vi "OP500ZP_CLUSTER_OCVACIR.vi"(10 "MESURES_OCVACIR":cluster{string, string, string}, 11 "Tableau 3":string[][](array[string])) -> (2 "Tableau":bool[](array[boolean]), 3 "Tableau 2":string[][](array[string]))   [LabVIEW 2020]
uses:
  VG/PackType.vi
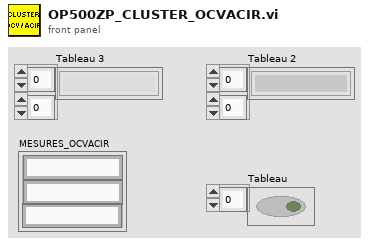
[diagram p1: front panel]
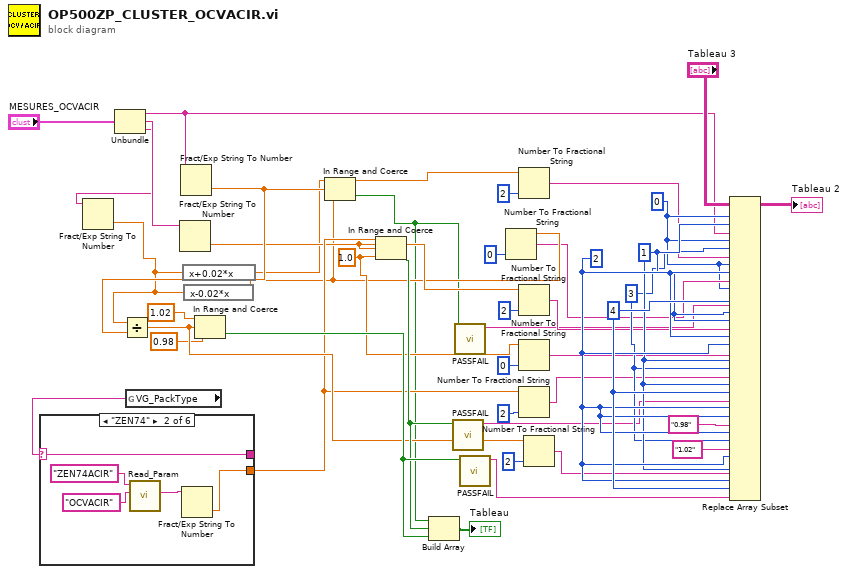
[diagram p0: block diagram]
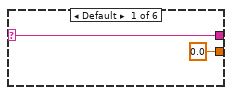
[diagram p2: hidden frame]
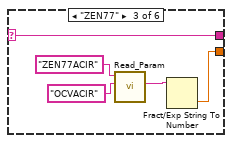
[diagram p3: hidden frame]
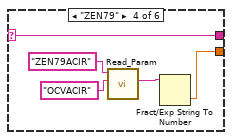
[diagram p4: hidden frame]
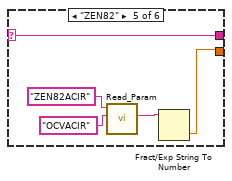
[diagram p5: hidden frame]
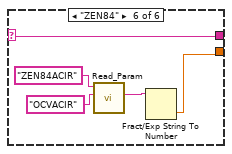
[diagram p6: hidden frame]
diagram:
  w20 = 1.0 ("limite inférieure")
  w37 = 2 ("disabled index (col)")
  w38 = 4 ("disabled index (col)")
  w34 = 3 ("disabled index (col)")
  w35 = 1 ("disabled index (col)")
  w11 = 0 ("index (row)")
  n1 = Unbundle("MESURES_OCVACIR") -> (w4:string, w3:string, w1:string)
  n2 = Fract/Exp String To Number(string=w1) -> (number=w2:dbl)  [unwired: 3 in, 1 out]
  n3 = global read "PackType.vi" "VG_PackType"() -> (w14:string)
  n4 = case shown="\"ZEN74\"" w14 {
    selector: w14 -> [w45 w50 w55 w60 w65 w70]
    tunnel: [w45 w50 w55 w60 w65 w70] -> _
    tunnel: [0.0 ("ZEN84ACIR") w46 w51 w56 w61 w66] -> w23
    frame Default {
    }
    frame "ZEN74" {
      n5 = call "Read_Param.vi"("section"="OCVACIR", "key"="ZEN74ACIR") -> ("str"=w49:string)  [unwired: 5 in, 4 out]
      n6 = Fract/Exp String To Number(string=w49) -> (number=w46:dbl)  [unwired: 3 in, 1 out]
    }
    frame "ZEN77" {
      n7 = call "Read_Param.vi"("section"="OCVACIR", "key"="ZEN77ACIR") -> ("str"=w54:string)  [unwired: 5 in, 4 out]
      n8 = Fract/Exp String To Number(string=w54) -> (number=w51:dbl)  [unwired: 3 in, 1 out]
    }
    frame "ZEN79" {
      n9 = call "Read_Param.vi"("section"="OCVACIR", "key"="ZEN79ACIR") -> ("str"=w59:string)  [unwired: 5 in, 4 out]
      n10 = Fract/Exp String To Number(string=w59) -> (number=w56:dbl)  [unwired: 3 in, 1 out]
    }
    frame "ZEN82" {
      n11 = call "Read_Param.vi"("section"="OCVACIR", "key"="ZEN82ACIR") -> ("str"=w64:string)  [unwired: 5 in, 4 out]
      n12 = Fract/Exp String To Number(string=w64) -> (number=w61:dbl)  [unwired: 3 in, 1 out]
    }
    frame "ZEN84" {
      n13 = call "Read_Param.vi"("section"="OCVACIR", "key"="ZEN84ACIR") -> ("str"=w69:string)  [unwired: 5 in, 4 out]
      n14 = Fract/Exp String To Number(string=w69) -> (number=w66:dbl)  [unwired: 3 in, 1 out]
    }
  }
  n15 = Fract/Exp String To Number(string=w3) -> (number=w18:dbl)  [unwired: 3 in, 1 out]
  n16 = Fract/Exp String To Number(string=w4) -> (number=w27:dbl)  [unwired: 3 in, 1 out]
  n17 = Divide(x=w2, y=w27) -> (x/y=w32:dbl)
  n18 = expression code="x+0.02*x"(w2) -> (w15:dbl)
  n19 = expression code="x-0.02*x"(w2) -> (w16:dbl)
  n20 = In Range and Coerce(upper limit=1.02 ("limite supérieure"), x=w32, lower limit=0.98 ("limite inférieure")) -> (In Range?=w41:bool)  [unwired: 1 out]
  n21 = In Range and Coerce(upper limit=w15, x=w27, lower limit=w16) -> (In Range?=w12:bool)  [unwired: 1 out]
  n22 = In Range and Coerce(upper limit=w23, x=w18, lower limit=w20) -> (In Range?=w40:bool)  [unwired: 1 out]
  n23 = Build Array(w12, w40, w41) -> (→"Tableau":bool[])
  n24 = call <vilib>:"PASSFAIL.vi"("E"=w40) -> ("S"=w26:string)  [unwired: 10 in]
  n25 = call <vilib>:"PASSFAIL.vi"("E"=w12) -> ("S"=w10:string)  [unwired: 10 in]
  n26 = call <vilib>:"PASSFAIL.vi"("E"=w41) -> ("S"=w39:string)  [unwired: 10 in]
  n27 = Number To Fractional String(number=w16, precision (6)=i16 0 ("précision (6)")) -> (F-format string=w13:string)  [unwired: 2 in]
  n28 = Number To Fractional String(number=w15, precision (6)=i16 2 ("précision (6)")) -> (F-format string=w9:string)  [unwired: 2 in]
  n29 = Number To Fractional String(number=w18, precision (6)=i16 2 ("précision (6)")) -> (F-format string=w19:string)  [unwired: 2 in]
  n30 = Number To Fractional String(number=w20, precision (6)=i16 0 ("précision (6)")) -> (F-format string=w21:string)  [unwired: 2 in]
  n31 = Number To Fractional String(number=w23, precision (6)=i16 2 ("précision (6)")) -> (F-format string=w25:string)  [unwired: 2 in]
  n32 = Number To Fractional String(number=w32, precision (6)=i16 2 ("précision (6)")) -> (F-format string=w33:string)  [unwired: 2 in]
  n33 = Replace Array Subset(array="Tableau 3", new element #1=w4, index (row) #1=w11, index (col) #1=w35, new element #2=w9, index (row) #2=w11, index (col) #2=w34, new element #3=w13, index (row) #3=w11, index (col) #3=w37, new element #4=w10, index (row) #4=w11, index (col) #4=w38, new element #5=w19, index (row) #5=w35, index (col) #5=w35, new element #6=w21, index (row) #6=w35, index (col) #6=w37, new element #7=w25, index (row) #7=w35, index (col) #7=w34, new element #8=w26, index (row) #8=w35, index (col) #8=w38, new element #9="0.98" ("nouvel élément/sous-tableau"), index (row) #9=w37, index (col) #9=w37, new element #10="1.02" ("nouvel élément/sous-tableau"), index (row) #10=w37, index (col) #10=w34, new element #11=w33, index (row) #11=w37, index (col) #11=w35, new element #12=w39, index (row) #12=w37, index (col) #12=w38) -> (→"Tableau 2":string[][])
